vi "Condition Name Actor.vi"(8 "error in":errorcluster, 9 "Terminals (All)":T4, 10 "Name Actor":T1) -> (0 "error out":errorcluster, 2 "Terminal Attributes (Init)":T2)   [LabVIEW 2025, in "_Rescript.lvlib" / "Actor.lvlib" / "Actor.lvclass"]
uses:
  Actor.lvclass
  Actor.lvclass/Actor.ctl
  _Rescript.lvlib
  Terminals.ctl
  Attributes.ctl
  Terminal Attributes.ctl
  Name Actor.ctl
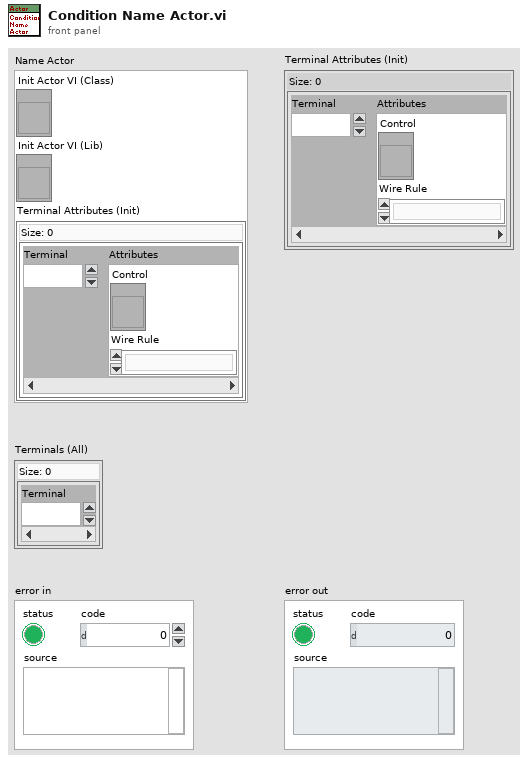
[diagram p1: front panel]
types:
  T1 = typedef "_Rescript.lvlib/Actor.lvlib/Actor.lvclass/Name Actor.ctl" = cluster{"Init Actor VI (Class)":refnum<vi>, "Init Actor VI (Lib)":refnum<vi>, "Terminal Attributes (Init)":T2}
  T2 = typedef "_Rescript.lvlib/Terminal Attributes.ctl" = map{i32, T3}
  T3 = typedef "_Rescript.lvlib/Attributes.ctl" = cluster{"Control":refnum<vi>, "Wire Rule":enum16{"Invalid Wire Rule", "Required", "Recommended", "Optional", "Dynamic Dispatch"}}
  T4 = typedef "_Rescript.lvlib/Terminals.ctl" = set{i32}
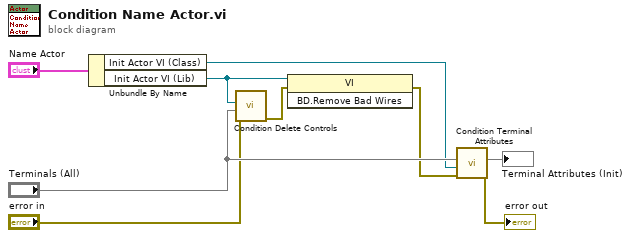
[diagram p0: block diagram]
diagram:
  n1 = Unbundle By Name("Name Actor") -> ("Init Actor VI (Class)"=w1:refnum<vi>, "Init Actor VI (Lib)"=w2:refnum<vi>)
  n2 = call "Condition Delete Controls.vi"("error in"="error in", "Terminals"="Terminals (All)", "VI"=w2) -> ("error out"=w8:errorcluster)  [unwired: 8 in]
  n3 = invoke class="VI" method="BD.Remove Bad Wires"(reference=w2, error in=w8) -> (error out=w5:errorcluster)  [unwired: 1 in, 2 out]
  n4 = call "Condition Terminal Attributes.vi"("error in"=w5, "VI"=w1, "Terminals"="Terminals (All)") -> ("error out"=→"error out":errorcluster, "Terminal Attributes"=→"Terminal Attributes (Init)":T2)  [unwired: 7 in]
